vi "Host.vi"() -> ()   [LabVIEW 2019]
uses:
  <vilib>/FPGAPlugInAG/PXIe-7915/niLvFpga_Open_PXIe-7915.vi
  <vilib>/rvi/interface/common/dynamic/niFpgaDynamicAddResources.vi
  <vilib>/Utility/error.llb/Error Cluster From Error Code.vi
  <vilib>/rvi/errors/niLvFpgaAdjustHostInterfaceError.vi
  <vilib>/FPGAPlugInAG/Dynamic/niLvFpga_Run_Dynamic.vi
  <vilib>/FPGAPlugInAG/Dynamic/niLvFpga_Close_Dynamic.vi
  <vilib>/rvi/interface/nirviOpenFPGA/nirviOpenFPGA.xnode
  FPGA Bitfiles/choleskyfpgav1_FPGATarget_Target2_qdS2-QLcSpk.lvbitx
  Target.vi
  <vilib>/rvi/interface/nirviReadWriteControl/nirviReadWriteControl.xnode
  <vilib>/rvi/interface/nirviMethod/nirviMethod.xnode
  <vilib>/rvi/interface/nirviCloseFPGA/nirviCloseFPGA.xnode
  <vilib>/rvi/interface/Simulation/niFpgaSimulationCallBeginRW.vi
  NiFpgaLv.dll
panel:
  in  "stop":bool
  out "sqrt(x)":sgl
  in  "Element":sgl=1.0
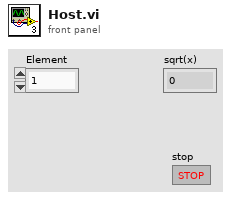
[diagram p1: front panel]
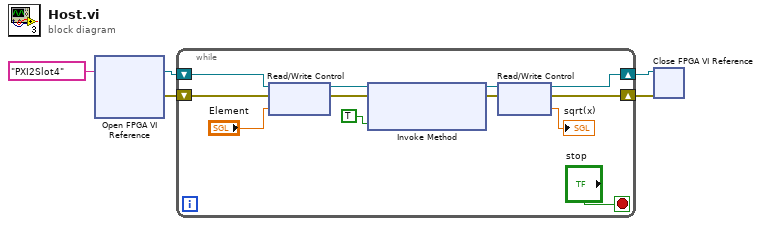
[diagram p0: block diagram]
diagram:
  n1 = xnode "Open FPGA VI Reference"("resource name"=tag "PXI2Slot4") -> ("FPGA VI Reference Out"=w5:refnum<k20>, "error out"=w3:errorcluster)  [unwired: 1 in]
  n2 = while {
    shift-right: [w14] -> w4
    shift-left: w5 -> [w17]
    shift-right: [w10] -> w2
    shift-left: w3 -> [w13]
    stop <- "stop" stop-if-true
    n3 = xnode "Read/Write Control"("FPGA VI Reference In"=w17, "error in"=w13, "Element"="Element") -> ("FPGA VI Reference Out"=w16:refnum<k20>, "error out"=w12:errorcluster)
    n4 = xnode "Invoke Method"("FPGA VI Reference In"=w16, "error in"=w12, "Wait Until Done (F)"=TRUE) -> ("FPGA VI Reference Out"=w15:refnum<k20>, "error out"=w11:errorcluster)
    n5 = xnode "Read/Write Control"("FPGA VI Reference In"=w15, "error in"=w11) -> ("FPGA VI Reference Out"=w14:refnum<k20>, "error out"=w10:errorcluster, "sqrt(x)"=→"sqrt(x)":sgl)
  }
  n6 = xnode "Close FPGA VI Reference"("FPGA VI Reference In"=w4, "error in"=w2) -> ()  [unwired: 1 out]
